vi "Query Metadata.vi"() -> ()   [LabVIEW 2024]
uses:
  <vilib>/Plug-In SDKs/Clients/Metadata Store V1/Metadata Store Client.lvlibp/API/Metadata Store V1/Query Operators.vi
  <vilib>/Plug-In SDKs/Clients/Metadata Store V1/Metadata Store Client.lvlibp/API/Metadata Store V1/Query Test Stations.vi
  <vilib>/Plug-In SDKs/Clients/Metadata Store V1/Metadata Store Client.lvlibp/API/Metadata Store V1/Query Hardware Items.vi
  <vilib>/Plug-In SDKs/Clients/Metadata Store V1/Metadata Store Client.lvlibp/API/Metadata Store V1/Query UUTs.vi
  <vilib>/Plug-In SDKs/Clients/Metadata Store V1/Metadata Store Client.lvlibp/API/Metadata Store V1/Query Software Items.vi
  <vilib>/Plug-In SDKs/Clients/Metadata Store V1/Metadata Store Client.lvlibp
panel:
  in  "Tab Control":T1(tab)
  out "Filtered operators (by role containing 'Test Engineer')":string[](array[string])
  out "Filtered test stations (by name starting with 'Test')":string[](array[string])
  out "Filtered hardware items (by model containing '4081')":string[](array[string])
  out "Filtered UUTs (by name ending with 'v1.3')":string[](array[string])
  out "Filtered software items (by product 'Python')":string[](array[string])
  out "error out":errorcluster
  # "Query Metadata\n\nThis VI provides examples of querying metadata items.\nRun Publish Data.vi to create data to query with this VI."
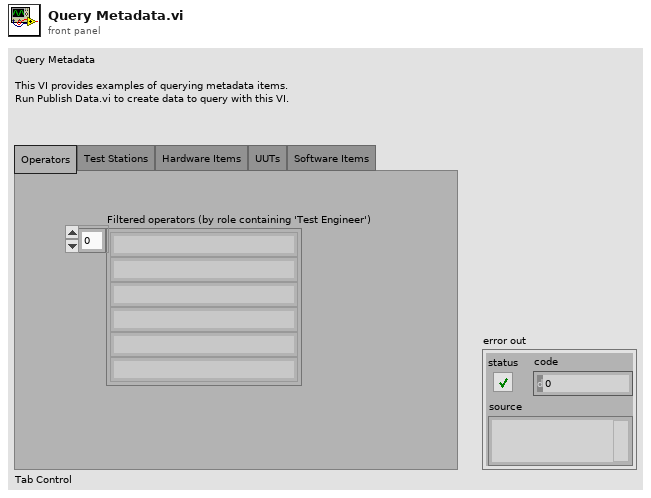
[diagram p1: front panel]
types:
  T1 = enum32{"Operators", "Test Stations", "Hardware Items", "UUTs", "Software Items"}
  T2 = typedef "NI Metadata Types.lvlib/Operator.ctl" = cluster{"operator name":string, "role":string, "id":string, "link":string, "extensions":T3[], "schema id":string}
  T3 = typedef "NI Metadata Types.lvlib/Extension.ctl" = cluster{"name":string, "value":string}
  T4 = typedef "NI Metadata Types.lvlib/Test Station.ctl" = cluster{"test station name":string, "asset identifier":string, "id":string, "link":string, "extensions":T3[], "schema id":string}
  T5 = typedef "NI Metadata Types.lvlib/UUT.ctl" = cluster{"model name":string, "family":string, "manufacturers":string[], "part number":string, "id":string, "link":string, "extensions":T3[], "schema id":string}
  T6 = typedef "NI Metadata Types.lvlib/Software Item.ctl" = cluster{"product":string, "version":string, "id":string, "link":string, "extensions":T3[], "schema id":string}
  T7 = typedef "NI Metadata Types.lvlib/Hardware Item.ctl" = cluster{"model":string, "manufacturer":string, "part number":string, "serial number":string, "calibration due date":string, "asset identifier":string, "id":string, "link":string, "extensions":T3[], "schema id":string}
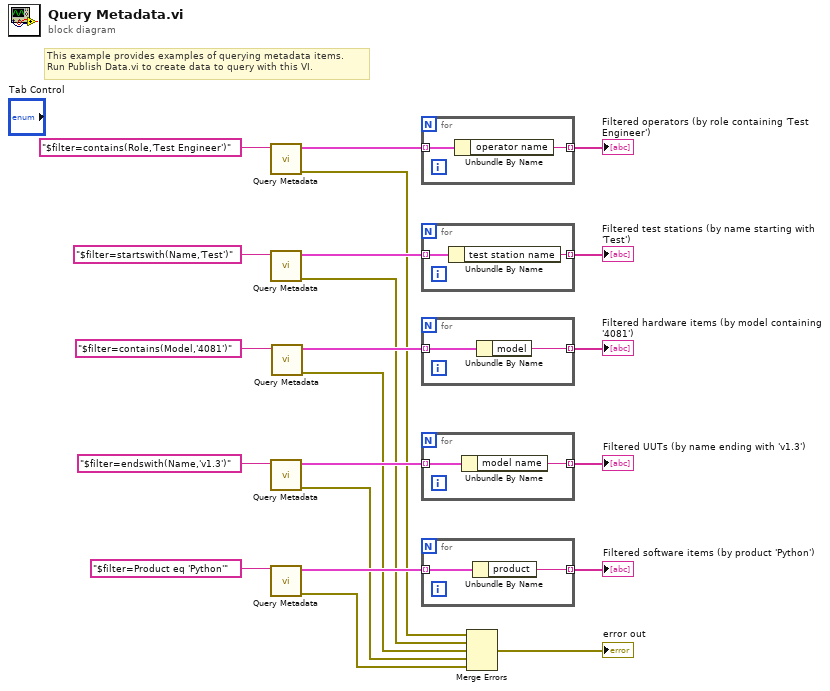
[diagram p0: block diagram]
diagram:
  # "This example provides examples of querying metadata items.\nRun Publish Data.vi to create data to query with this VI."
  n1 = call-poly <vilib>:"Query Metadata.vi"("odata query"="$filter=contains(Role,'Test Engineer')") -> ("error out"=w6:errorcluster, "operators"=w20:T2[])  [unwired: 9 in]
  n2 = call-poly <vilib>:"Query Metadata.vi"("odata query"="$filter=startswith(Name,'Test')") -> ("error out"=w5:errorcluster, "test stations"=w17:T4[])  [unwired: 9 in]
  n3 = call-poly <vilib>:"Query Metadata.vi"("odata query"="$filter=endswith(Name,'v1.3')") -> ("error out"=w3:errorcluster, "uuts"=w11:T5[])  [unwired: 9 in]
  n4 = call-poly <vilib>:"Query Metadata.vi"("odata query"="$filter=Product eq 'Python'") -> ("error out"=w2:errorcluster, "software items"=w8:T6[])  [unwired: 9 in]
  n5 = call-poly <vilib>:"Query Metadata.vi"("odata query"="$filter=contains(Model,'4081')") -> ("error out"=w4:errorcluster, "hardware items"=w14:T7[])  [unwired: 9 in]
  n6 = for {
    tunnel: w20 -> [w23] mode=indexing
    tunnel: [w22] -> w19 mode=indexing
    n7 = Unbundle By Name(w23) -> ("operator name"=w22:string)
  }
  "Filtered operators (by role containing 'Test Engineer')" <- w19
  n8 = for {
    tunnel: w17 -> [w25] mode=indexing
    tunnel: [w24] -> w16 mode=indexing
    n9 = Unbundle By Name(w25) -> ("test station name"=w24:string)
  }
  "Filtered test stations (by name starting with 'Test')" <- w16
  n10 = for {
    tunnel: w14 -> [w27] mode=indexing
    tunnel: [w26] -> w15 mode=indexing
    n11 = Unbundle By Name(w27) -> ("model"=w26:string)
  }
  "Filtered hardware items (by model containing '4081')" <- w15
  n12 = for {
    tunnel: w11 -> [w29] mode=indexing
    tunnel: [w28] -> w10 mode=indexing
    n13 = Unbundle By Name(w29) -> ("model name"=w28:string)
  }
  "Filtered UUTs (by name ending with 'v1.3')" <- w10
  n14 = for {
    tunnel: w8 -> [w31] mode=indexing
    tunnel: [w30] -> w9 mode=indexing
    n15 = Unbundle By Name(w31) -> ("product"=w30:string)
  }
  "Filtered software items (by product 'Python')" <- w9
  n16 = Merge Errors(w6, w5, w4, w3, w2) -> (→"error out":errorcluster)
